vi "Encode 2D String to Support Multiline.vi"(6 "Characters to Encode":string[](array[string])=[",", "\"", "\n"], 8 "error in (no error)":errorcluster, 11 "2D Array In":string[][](array[string])) -> (0 "error out":errorcluster, 3 "2D Array Out":string[][](array[string]))   [LabVIEW 2016, in "SLL Spreadsheet.lvlib"]
doc: "This VI encodes a 2D String array similar to how Excel does, when a cell contains new line character, comma or double quotes."
uses:
  SLL Spreadsheet.lvlib
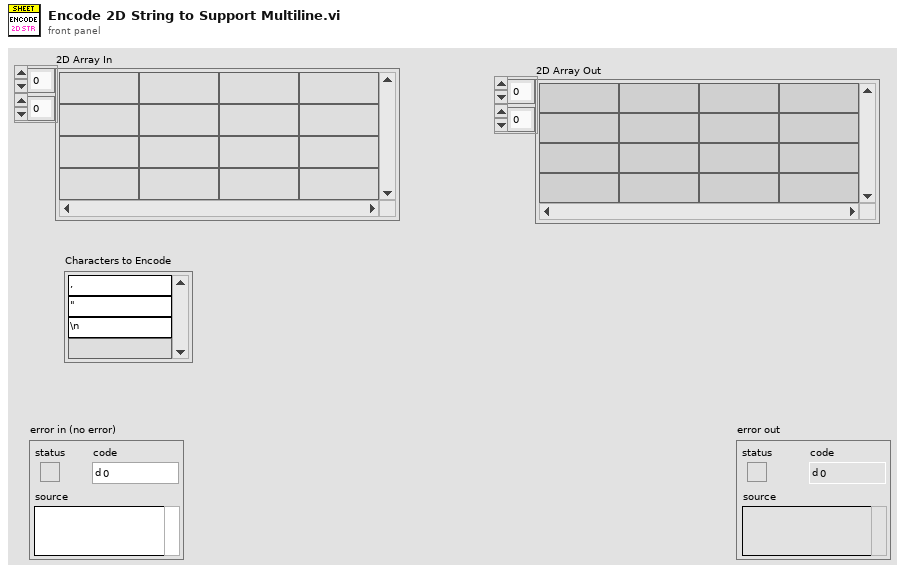
[diagram p1: front panel]
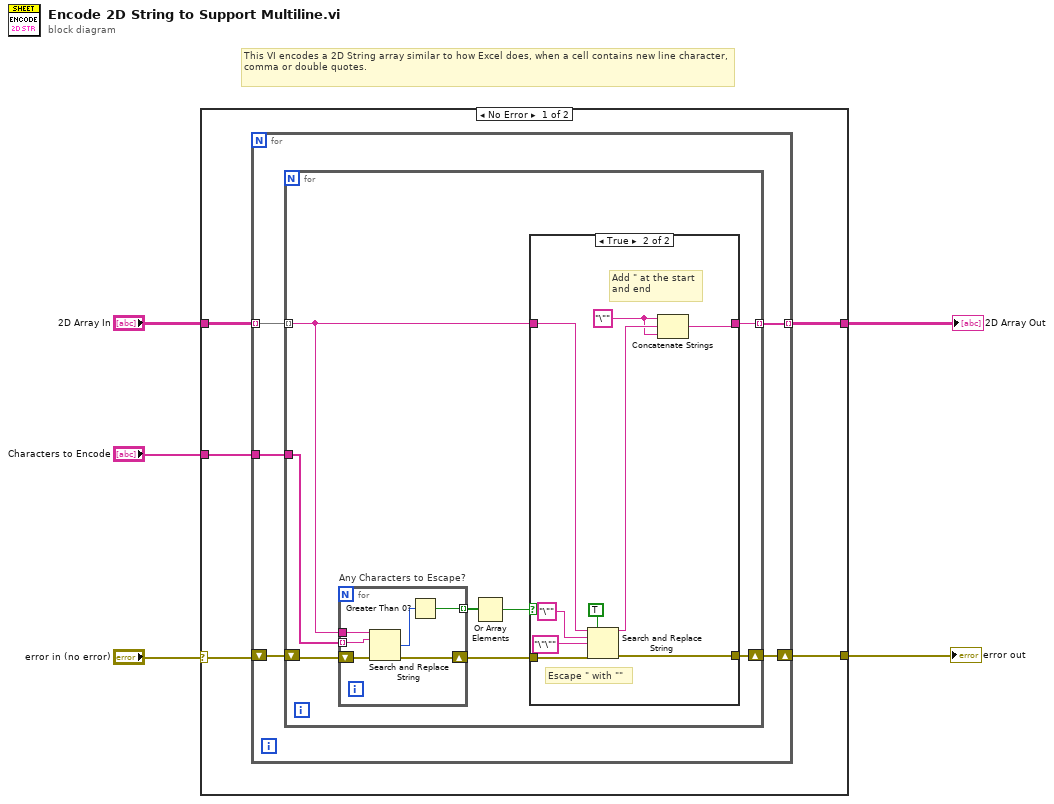
[diagram p0: block diagram]
diagram:
  # "This VI encodes a 2D String array similar to how Excel does, when a cell contains new line character, comma or double quotes."
  n1 = case shown="No Error" "error in (no error)" {
    selector: "error in (no error)" -> [w8 w41]
    tunnel: "2D Array In" -> [w10 _]
    tunnel: [w9 _] -> w4
    tunnel: [w7 w41] -> w2
    tunnel: "Characters to Encode" -> [w6 _]
    frame No Error {
      n2 = for {
        tunnel: w10 -> [w15] mode=indexing
        tunnel: [w14] -> w9 mode=indexing
        tunnel: w6 -> [w13]
        shift-right: [w11] -> w7
        shift-left: w8 -> [w12]
        n3 = for {
          tunnel: w15 -> [w17] mode=indexing
          tunnel: [w19] -> w14 mode=indexing
          tunnel: w13 -> [w23]
          shift-right: [w16] -> w11
          shift-left: w12 -> [w22]
          n4 = for "Any Characters to Escape?" {
            tunnel: w17 -> [w40]
            tunnel: w23 -> [w39] mode=indexing
            tunnel: [w36] -> w21 mode=indexing
            shift-right: [w35] -> w18
            shift-left: w22 -> [w38]
            n5 = Search and Replace String(input string=w40, search string=w39, error in=w38) -> (number of replacements=w37:i32, error out=w35:errorcluster)  [unwired: 5 in, 2 out]
            n6 = Greater Than 0?(x=w37) -> (x > 0?=w36:bool)
          }
          n7 = Or Array Elements(Boolean array=w21) -> (logical OR=w20:bool)
          n8 = case shown="True" w20 {
            tunnel: w17 -> [w25 w30]
            tunnel: [w25 w27] -> w19
            tunnel: w18 -> [w24 w34]
            tunnel: [w24 w26] -> w16
            frame False {
            }
            frame True {
              w28 = "\"" ("string")
              # "Add \" at the start\nand end"
              # "Escape \" with \"\""
              n9 = Search and Replace String(replace all?=TRUE ("replace all? (F)"), input string=w30, search string="\"" ("input string"), replace string="\"\"" ("input string"), error in=w34) -> (result string=w29:string, error out=w26:errorcluster)  [unwired: 3 in, 2 out]
              n10 = Concatenate Strings(w28, w29, w28) -> (w27:string)
            }
          }
        }
      }
    }
    frame Error {
    }
  }
  "2D Array Out" <- w4
  "error out" <- w2
